vi "OpenImg_WithVisionInfor.vi"(2 "Image Name":string, 3 "Template File Path":path) -> (0 "can't find template?":bool, 1 "Image Out":T1)   [LabVIEW 2014]
uses:
  <vilib>/vision/Image Controls.llb/IMAQ Image.ctl
panel:
  out "error out":errorcluster
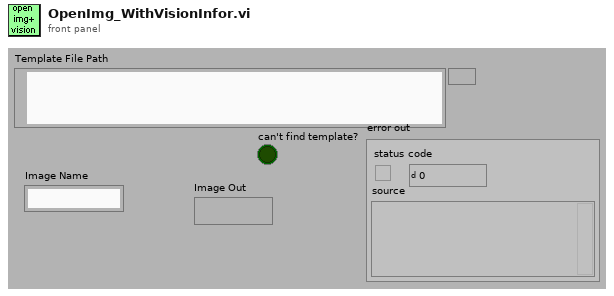
[diagram p1: front panel]
types:
  T1 = typedef "IMAQ Image.ctl" = refnum<image>
  T2 = typedef "Image Type" = u32
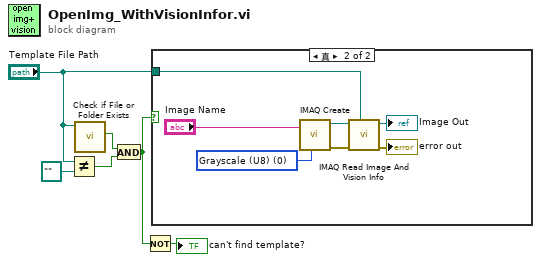
[diagram p0: block diagram]
diagram:
  n1 = Not Equal?(x="Template File Path", y=path "") -> (x != y?=w4:bool)
  n2 = call <vilib>:"Check if File or Folder Exists.vi"("path"="Template File Path") -> ("file or folder exists?"=w5:bool)  [unwired: 8 in, 2 out]
  n3 = And(x=w5, y=w4) -> (x .and. y?=w2:bool)
  n4 = Not(x=w2) -> (.not. x?=→"can't find template?":bool)
  n5 = case shown="真" w2 {
    tunnel: "Template File Path" -> [_ w7]
    frame False {
    }
    frame True {
      w9 = T2 0 items=["Grayscale (U8)", "Grayscale (I16)", "Grayscale (SGL)", "Complex (CSG)", "RGB (U32)", "HSL (U32)", "RGB (U64)", "Grayscale (U16)"] ("Image Type")
      n6 = call "IMAQ Create"("Image Name"="Image Name", "Image Type"=w9) -> ("New Image"=w10:T1, "error out"=w11:errorcluster)  [unwired: 2 in, 1 out]
      n7 = call "IMAQ Read Image And Vision Info"("File Path"=w7, "error in (no error)"=w11, "Image"=w10) -> ("error out"=→"error out":errorcluster, "Image Out"=→"Image Out":T1)  [unwired: 1 in, 6 out]
    }
  }
